vi "ZZZ un horror Chroma 1905x Series Get Configuration POP.vi"(0 "inst handle in":refnum<visa-resource-name>, 3 "error in":T1) -> (5 "inst handle out":refnum<visa-resource-name>, 8 "error out":T1)   [LabVIEW 2025]
doc: "Contact Chroma\nTEL: +886-2-2298-3855 \nTEL: +886-3-397-5788 \nFAX: +886-2-2298-3596\nFAX: +886-3-327-4703 \nURL: http://www.chromaate.com \nE-mail: chroma@chroma.com.tw"
panel:
  out "Channels Low":string
  out "Channels High":string
  out "Ramp Time":string
  out "Test Time":string
  out "Arc Detection Limit":string
  out "Low Limit":string
  out "Mode":string
  out "Hi Limit":string
  out "Voltage Level":string
  in  "Step Number":dbl=1.0 min=1.0 max=25.0 step=1.0
  in  "Finished":bool
  in  "Configure":bool
  # "Configuration Screen"
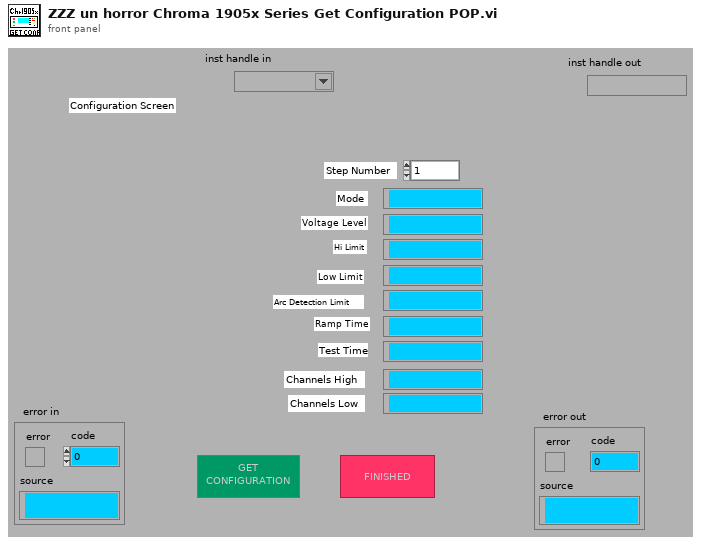
[diagram p1: front panel]
types:
  T1 = cluster{"error":bool, "code":i8, "source":string}
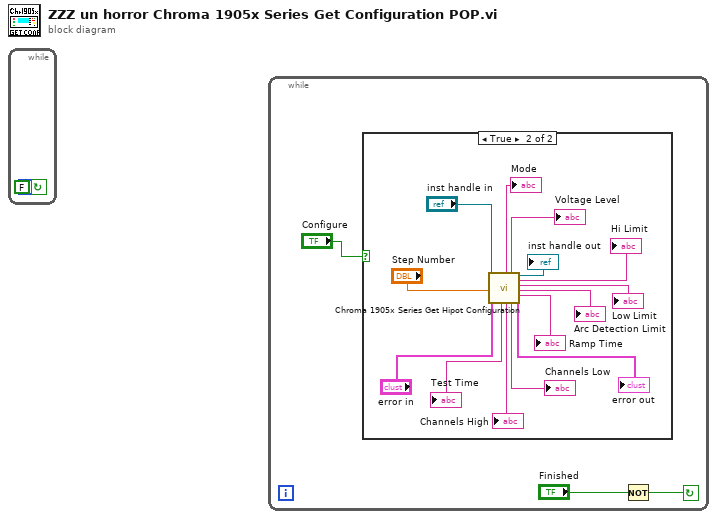
[diagram p0: block diagram]
diagram:
  n1 = while {
    stop <- FALSE continue-if-true
  }
  n2 = while {
    stop <- w2 continue-if-true
    n3 = case shown="True" "Configure" {
      frame False {
      }
      frame True {
        n4 = call "Chroma 1905x Series Get Hipot Configuration.vi"("inst handle in"="inst handle in", "Step Number"="Step Number", "error in"="error in") -> ("Test Time"=→"Test Time":string, "Mode"=→"Mode":string, "Channels High"=→"Channels High":string, "Voltage Level"=→"Voltage Level":string, "Channels Low"=→"Channels Low":string, "inst handle out"=→"inst handle out":refnum<visa-resource-name>, "Hi Limit"=→"Hi Limit":string, "Low Limit"=→"Low Limit":string, "Arc Detection Limit"=→"Arc Detection Limit":string, "Ramp Time"=→"Ramp Time":string, "error out"=→"error out":T1)  [unwired: 5 in, 1 out]
      }
    }
    n5 = Not(x="Finished") -> (.not. x?=w2:bool)
  }
